vi "Main PDF REPORT Python Code.vi"(0 "File Path":string, 5 "X axis":string="Time(Sec)", 7 "Y AXIS":string="Normal Load (N),Friction Force(N),Coefficient of Friction, Depth (Microns)", 9 "organization":string="Paltro Systems", 11 "error in (no error)":errorcluster, 12 "Revision":string="\"Rev A\"") -> (15 "error out":errorcluster)   [LabVIEW 2025]
panel:
  out "return value":string
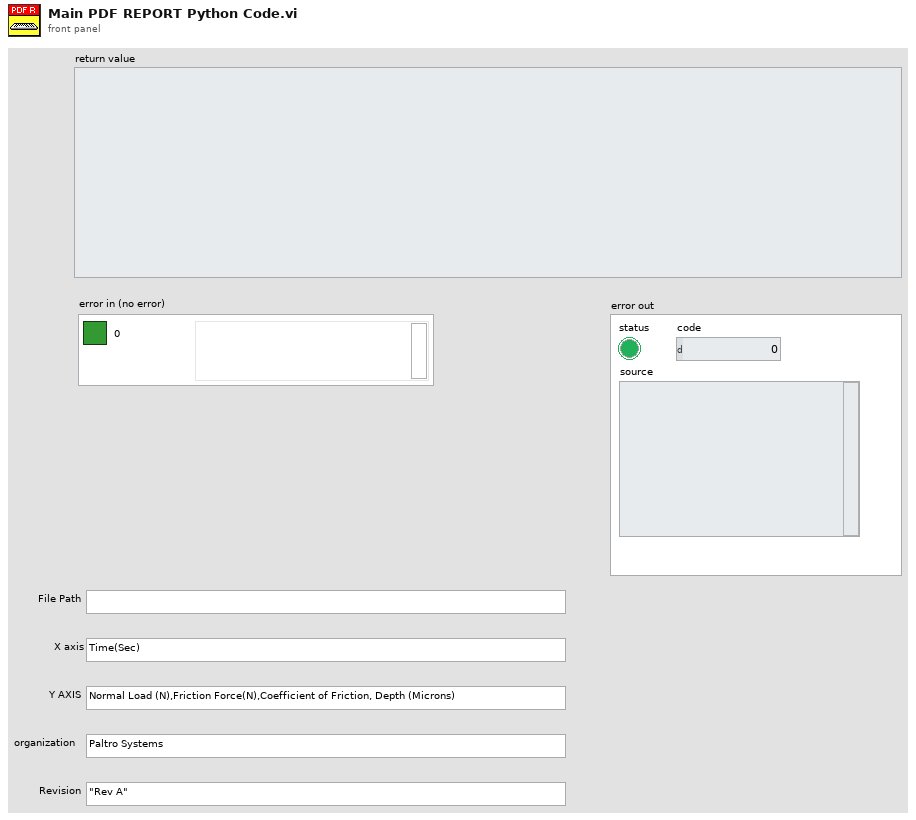
[diagram p1: front panel]
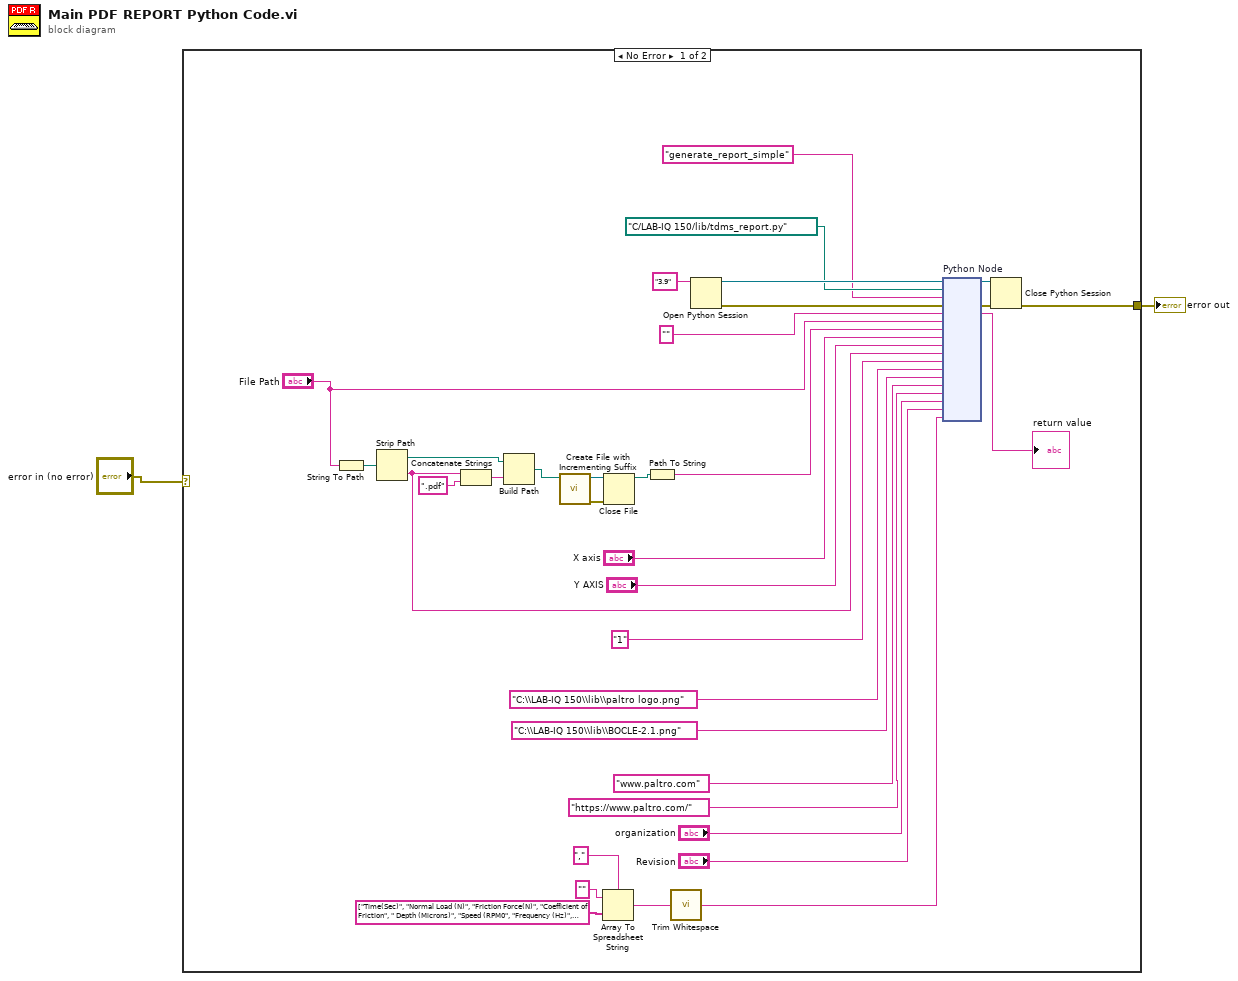
[diagram p0: block diagram]
diagram:
  n1 = case shown="No Error" "error in (no error)" {
    tunnel: [w8 _] -> w2
    frame No Error {
      n2 = String To Path(string="File Path") -> (path=w17:path)
      n3 = Strip Path(path=w17) -> (stripped path=w14:path, name=w9:string)
      n4 = Concatenate Strings(w9, ".pdf" ("string")) -> (w15:string)
      n5 = Build Path(base path=w14, name or relative path=w15) -> (appended path=w13:path)
      n6 = call <vilib>:"Create File with Incrementing Suffix.vi"("file path"=w13) -> ("error out"=w11:errorcluster, "refnum out"=w12:refnum<file>)  [unwired: 8 in, 1 out]
      n7 = Array To Spreadsheet String(delimiter (Tab)=",", array=string[] ["Time(Sec)", "Normal Load (N)", "Friction Force(N)", "Coefficient of Friction", " Depth (Microns)", "Speed (RPM0", "Frequency (Hz)", "Angle (Degree)", "Cyclic Friction Force (N)", "Cyclic Co-Efficient Friction Force", "Stage Temperature (Degree celcius)", "Sample Temperature (Degree celcius)", "Stroke Length (mm)", "Scratch Speed (mm/sec)", "Amb Humidity (%Rh)", "Amb Temperature (Deg C)", "Acoustic (mV)", "Mx(Nm)", "My(Nm)", "Mz (Nm)", "Humidity(%Rh)", "Sliding Distance (mm)", "Wear Track Diameter(mm)", "Fx(N)", "Fy(N)", "MTM Ball Speed(RPM)", "MTM Disc Speed (RPM)", "Entrainment Speed", "Slide Role", "Slip(%)", "Rotart Speed (m/sec)", "MTM Ball Speed (m/sec)", "MTM Disc Speed (m/sec)", "ECR (ohms)"], 3:"" ("format string")) -> (spreadsheet string=w4:string)
      n8 = Close File(refnum=w12, error in=w11) -> (path=w10:path)  [unwired: 1 out]
      n9 = Path To String(path=w10) -> (string=w32:string)
      n10 = call <vilib>:"Trim Whitespace.vi"("string"=w4) -> ("trimmed string"=w3:string)  [unwired: 1 in]
      n11 = Open Python Session(python version="3.9" ("Python version")) -> (session out=w36:refnum<k35>, error out=w34:errorcluster)  [unwired: 2 in]
      n12 = node "Python Node"(w36, path "C:/LAB-IQ 150/lib/tdms_report.py" ("module path"), "generate_report_simple" ("function name"), w34, "", "File Path", w32, "X axis", "Y AXIS", w9, "1" ("Python version"), "C:\\LAB-IQ 150\\lib\\paltro logo.png" ("LEFT HEADER ICON PATH"), "C:\\LAB-IQ 150\\lib\\BOCLE-2.1.png" ("Python version"), "www.paltro.com" ("Python version"), "https://www.paltro.com/" ("Python version"), "organization", "Revision", w3) -> (w28:refnum<k35>, w29:errorcluster, →"return value":string)  [unwired: 13 in, 2 out]
      n13 = Close Python Session(session in=w28, error in=w29) -> (11:w8:errorcluster)
    }
    frame Error {
    }
  }
  "error out" <- w2
